vi "test_TwoSessTwoPinTwoInstrTwoSiteReservation_CallNiFgenGetConnectionsNPinsMConnections_ReturnsThreeConnections.vi"(8 "error in":errorcluster) -> (0 "error out":errorcluster, 2 "result":string, 3 "pass":bool)   [LabVIEW 2020, in "MeasurementServerTests.lvlib"]
uses:
  MeasurementServerTests.lvlib
  Runtime/Clients/Session Management V1/Session Reservation/Connection.ctl
  Runtime/Clients/Session Management V1/Session Reservation/Session Reservation.lvclass
  03fc85e1-696b-4ece-a78b-f41470766ac0.vi
  a536e905-e99b-4ce6-9f7b-add65bd26abc.vi
  f2d0f46c-20cf-4e81-b3a3-5c4fc317eda1.vi
  Runtime/Sessions/niFGEN/NI Session Management niFGEN.lvlib
  Runtime/Sessions/niFGEN/Get Connections - NPin MConn.vi
  Runtime/Sessions/niFGEN/Connection with Session.ctl
  df021878-7cb2-419c-a41b-3322d3f1e455.vi
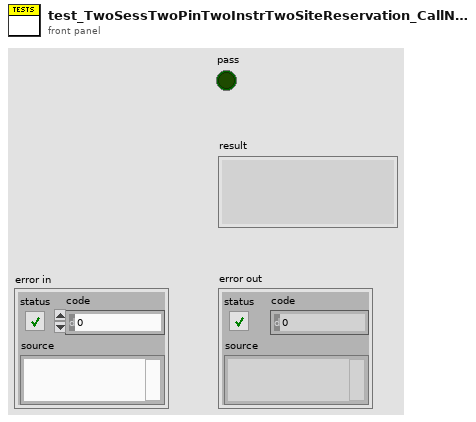
[diagram p1: front panel]
types:
  T1 = typedef "NI Session Management V1 Client.lvlib/Session Reservation.lvclass/Connection.ctl" = cluster{"pin or relay name":string, "site":i32, "instrument type id":string, "channel":string}
  T2 = typedef "NI Session Management niFGEN.lvlib/Connection with Session.ctl" = cluster{"connection":T1, "session":refnum<k15>}
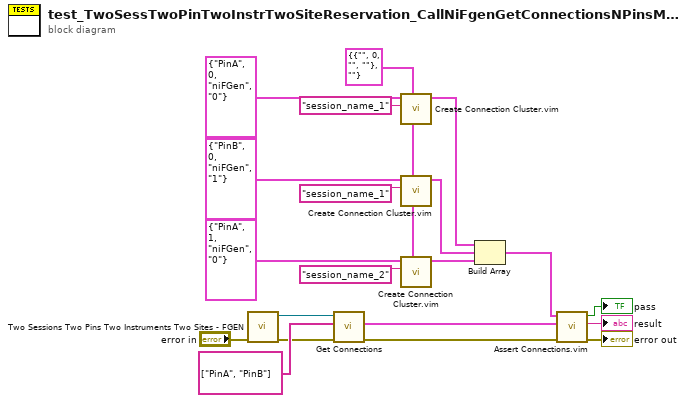
[diagram p0: block diagram]
diagram:
  w10 = T2 {"connection"={"pin or relay name"="", "site"=0, "instrument type id"="", "channel"=""}, "session"=""} ("niDCPower connection")
  n1 = call "Two Sessions Two Pins Two Instruments Two Sites - FGEN.vi"("error in"="error in") -> ("error out"=w4:errorcluster, "session reservation out"=w3:refnum<class "Session Reservation.lvclass">)  [unwired: 9 in]
  n2 = call-poly "Get Connections.vi"("error in"=w4, "pin or relay names"=string[] ["PinA", "PinB"], "session reservation in"=w3) -> ("error out"=w2:errorcluster, "connections"=w20:T2[])  [unwired: 6 in, 1 out]
  n3 = call "Create Connection Cluster.vim"("connection type"=w10, "session in"="session_name_1", "hardware independent connection in"=T1 {"pin or relay name"="PinA", "site"=0, "instrument type id"="niFGen", "channel"="0"} ("connection")) -> ("connection out"=w15:T2)  [unwired: 8 in]
  n4 = call "Create Connection Cluster.vim"("connection type"=w10, "session in"="session_name_1", "hardware independent connection in"=T1 {"pin or relay name"="PinB", "site"=0, "instrument type id"="niFGen", "channel"="1"} ("connection")) -> ("connection out"=w14:T2)  [unwired: 8 in]
  n5 = call "Create Connection Cluster.vim"("connection type"=w10, "session in"="session_name_2", "hardware independent connection in"=T1 {"pin or relay name"="PinA", "site"=1, "instrument type id"="niFGen", "channel"="0"} ("connection")) -> ("connection out"=w9:T2)  [unwired: 8 in]
  n6 = Build Array(w15, w14, w9) -> (w13:T2[])
  n7 = call "Assert Connections.vim"("error in"=w2, "actual connections"=w20, "expected connections"=w13) -> ("error out"=→"error out":errorcluster, "result"=→"result":string, "pass"=→"pass":bool)  [unwired: 6 in]
